vi "positioner_typedef.vi"(8 "error in":errorcluster, 9 "Array":dbl[](array[numeric]), 10 "command":string, 11 "reference in":refnum<vi>) -> (0 "error out":errorcluster)   [LabVIEW 2010]
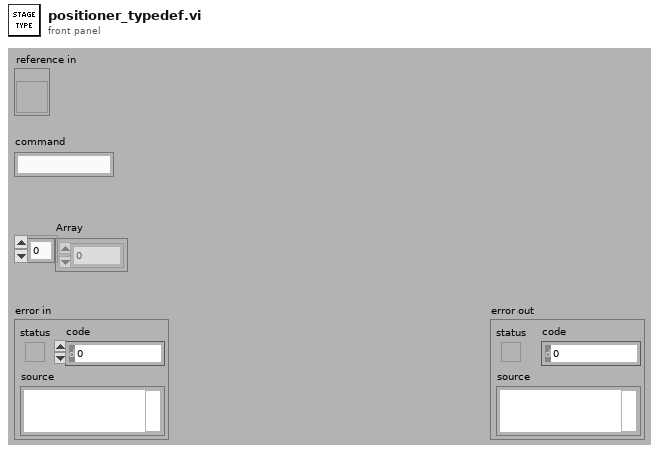
[diagram p1: front panel]
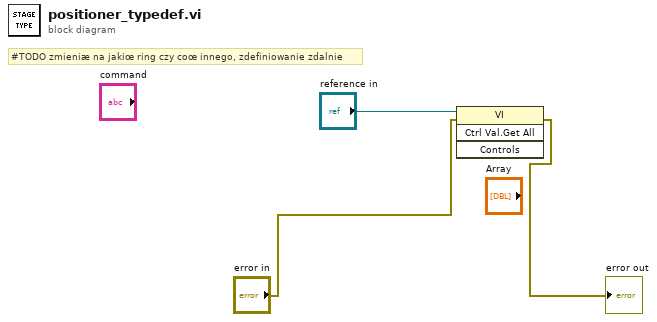
[diagram p0: block diagram]
diagram:
  # "#TODO zmieniæ na jakiœ ring czy coœ innego, zdefiniowanie zdalnie"
  n1 = invoke class="VI" method="Ctrl Val.Get All"(reference="reference in", error in="error in") -> (error out=→"error out":errorcluster)  [unwired: 2 in, 3 out]
